vi "emi_VI Bottom Panes Background.vi"(0 "VI Refnum(This VI)":refnum<vi>, 1 "Width(Screen)":i32=-1, 2 "Height(Screen)":i32=-1, 3 "Dark(Black)":u32(colorbox), 4 "Light(White)":u32(colorbox)=16448250, 5 "error in":errorcluster, 6 "Graphic Type(Flat Color)":T1) -> (14 "VI Refnum out":refnum<vi>, 19 "error IO":errorcluster)   [LabVIEW 2011]
doc: "Set the background graphic for the panes not touching the top edge"
uses:
  0 - General/Graphix/Private/emi_List Of Graphix.ctl
  <vilib>/picture/picture.llb/imagedata.ctl
  0 - General/Graphix/emi_BW 8Bit image to Linear DuoTone.vi
  0 - General/Graphix/emi_Tile Gradient Image.vi
  <vilib>/picture/picture.llb/Draw Flattened Pixmap.vi
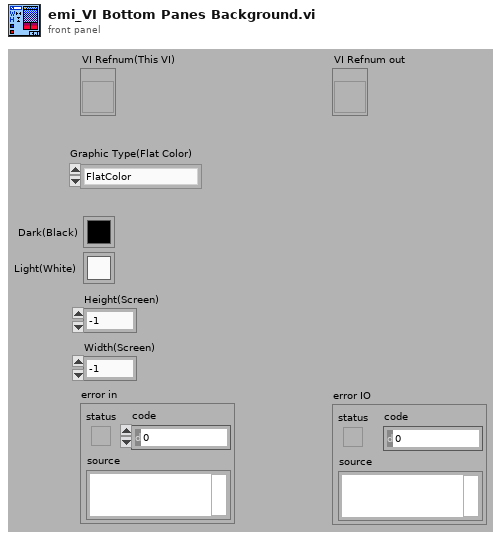
[diagram p1: front panel]
types:
  T1 = typedef "emi_List Of Graphix.ctl" = enum16{"FlatColor", "SharpGrad", "ShallowGrad", "GlasGradBord", "GlasGrad", "GlasGradBord 2"}
  T2 = typedef "imagedata.ctl" = cluster{"image type":i32, "image depth":i32, "image":u8[], "mask":u8[], "colors":u32[], "Rectangle":cluster{"left":i16, "top":i16, "right":i16, "bottom":i16}}
  T3 = typedef "LVRectTypeDef.ctl" = cluster{"left":i16, "top":i16, "right":i16, "bottom":i16}
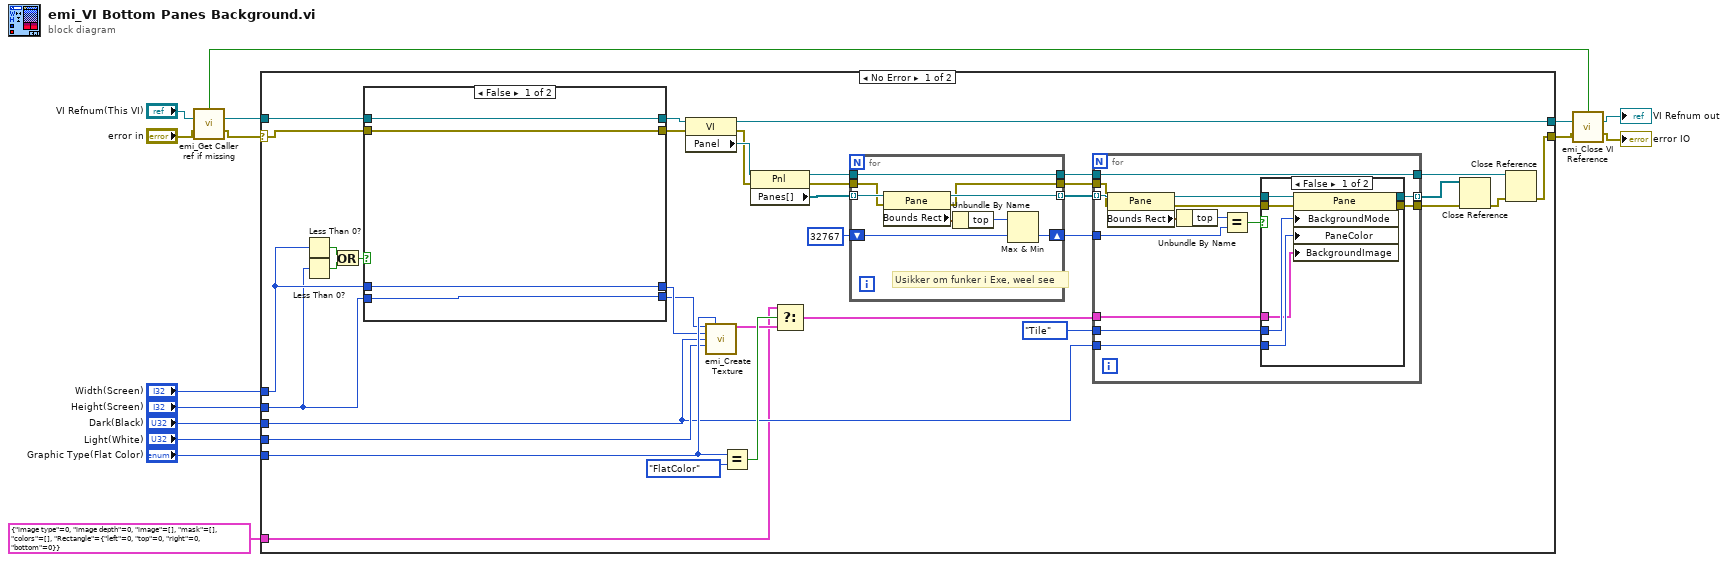
[diagram p0: block diagram]
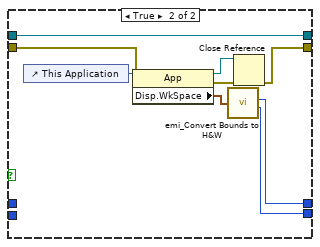
[diagram p3: hidden frame]
diagram:
  n1 = call "emi_Get Caller ref if missing.vi"("VI Refnum(Calling VI)"="VI Refnum(This VI)", "error in (no error)"="error in") -> ("Ref Generated"=w9:bool, "VI Refnum Out"=w1:refnum<vi>, "error out"=w4:errorcluster)  [unwired: 11 in]
  n2 = case shown="No Error" w4 {
    selector: w4 -> [w42 w98]
    tunnel: "Graphic Type(Flat Color)" -> [w50 _]
    tunnel: T2 {"image type"=0, "image depth"=0, "image"=[], "mask"=[], "colors"=[], "Rectangle"={"left"=0, "top"=0, "right"=0, "bottom"=0}} ("Image Data Out") -> [w33 _]
    tunnel: "Width(Screen)" -> [w45 _]
    tunnel: "Height(Screen)" -> [w44 _]
    tunnel: "Dark(Black)" -> [w35 _]
    tunnel: "Light(White)" -> [w49 _]
    tunnel: [w28 w98] -> w6
    tunnel: [w29 w97] -> w8
    tunnel: w1 -> [w26 w97]
    frame No Error {
      n3 = Less Than 0?(x=w45) -> (x < 0?=w46:bool)
      n4 = Less Than 0?(x=w44) -> (x < 0?=w47:bool)
      n5 = Or(x=w46, y=w47) -> (x .or. y?=w43:bool)
      n6 = case shown="False" w43 {
        tunnel: w42 -> [w87 w95]
        tunnel: [w87 w89] -> w37
        tunnel: w45 -> [w86 _]
        tunnel: [w86 w93] -> w41
        tunnel: w44 -> [w85 _]
        tunnel: [w85 w92] -> w40
        tunnel: [w84 w88] -> w27
        tunnel: w26 -> [w84 w88]
        frame False {
        }
        frame True {
          n7 = control-ref of="This Application"() -> (w96:refnum<vi>)
          n8 = property class="App"(reference=w96, error in=w95) -> (reference out=w90:refnum<vi>, error out=w91:errorcluster, "Disp.WkSpace"=w94:T3)
          n9 = call "emi_Convert Bounds to H&W.vi"("Bounds"=w94) -> ("Width"=w93:i32, "Height"=w92:i32)  [unwired: 6 in]
          n10 = Close Reference(reference=w90, error in (no error)=w91) -> (error out=w89:errorcluster)
        }
      }
      n11 = property class="VI"(reference=w27, error in=w37) -> (reference out=w29:refnum<vi>, error out=w38:errorcluster, "Panel"=w39:refnum<vi>)
      n12 = call "emi_Create Texture.vi"("Height(600)"=w40, "Graphic Type(Flat Color)"=w50, "Width(400)"=w41, "Dark(Black)"=w35, "Light(White)"=w49) -> ("Image Data Out"=w34:T2)  [unwired: 8 in, 2 out]
      n13 = Equal?(x=w50, y=emi_List_Of_Graphix."FlatColor" ("Graphic Type")) -> (x = y?=w48:bool)
      n14 = property class="Pnl"(reference=w39, error in=w38) -> (reference out=w23:refnum<vi>, error out=w22:errorcluster, "Panes[]"=w21:refnum<vi>[])
      n15 = Select(t=w33, s=w48, f=w34) -> (s? t:f=w32:T2)
      n16 = for {
        tunnel: w23 -> [w60]
        tunnel: w22 -> [w58]
        tunnel: w21 -> [w59] mode=indexing
        tunnel: [w57] -> w20 mode=indexing
        tunnel: [w60] -> w19
        tunnel: [w56] -> w18
        shift-right: [w52] -> w16
        shift-left: i16 32767 ("top") -> [w53]
        # "Usikker om funker i Exe, weel see"
        n17 = property class="Pane"(reference=w59, error in=w58) -> (reference out=w57:refnum<vi>, error out=w56:errorcluster, "Bounds Rect"=w55:T3)
        n18 = Unbundle By Name(w55) -> ("top"=w54:i16)
        n19 = Max & Min(x=w54, y=w53) -> (min(x,y)=w52:i16)  [unwired: 1 out]
      }
      n20 = for {
        tunnel: w20 -> [w67] mode=indexing
        tunnel: w18 -> [w66]
        tunnel: enum16{"Stretch", "Center", "Tile"}."Tile" ("Background Mode") -> [w74]
        tunnel: w35 -> [w73]
        tunnel: w32 -> [w72]
        tunnel: [w71] -> w24 mode=indexing
        tunnel: [w70] -> w25
        tunnel: w19 -> [w69]
        tunnel: [w69] -> w30
        tunnel: w16 -> [w63]
        n21 = property class="Pane"(reference=w67, error in=w66) -> (reference out=w65:refnum<vi>, error out=w62:errorcluster, "Bounds Rect"=w68:T3)
        n22 = Unbundle By Name(w68) -> ("top"=w64:i16)
        n23 = Equal?(x=w64, y=w63) -> (x = y?=w61:bool)
        n24 = case shown="False" w61 {
          tunnel: w74 -> [w81 _]
          tunnel: w73 -> [w80 _]
          tunnel: w72 -> [w79 _]
          tunnel: [w78 w83] -> w71
          tunnel: [w77 w82] -> w70
          tunnel: w65 -> [w76 w83]
          tunnel: w62 -> [w75 w82]
          frame False {
            n25 = property class="Pane"(reference=w76, error in=w75, "BackgroundMode"=w81, "PaneColor"=w80, "BackgroundImage"=w79) -> (reference out=w78:refnum<vi>, error out=w77:errorcluster)
          }
          frame True {
          }
        }
      }
      n26 = Close Reference(reference=w24, error in (no error)=w25) -> (error out=w31:errorcluster)
      n27 = Close Reference(reference=w30, error in (no error)=w31) -> (error out=w28:errorcluster)
    }
    frame Error {
    }
  }
  n28 = call "emi_Close VI Reference.vi"("Close ref?(T)"=w9, "VI Refnum"=w8, "error in (no error)"=w6) -> ("VI Refnum Out"=→"VI Refnum out":refnum<vi>, "error out"=→"error IO":errorcluster)  [unwired: 11 in]
